vi "MaxEye_ATE_Save_Configuration to File.vi"(0 "file path (use dialog)":path, 5 "Variant":variant, 7 "Config Header":string, 11 "error in (no error)":errorcluster) -> (15 "error out":errorcluster)   [LabVIEW 2021]
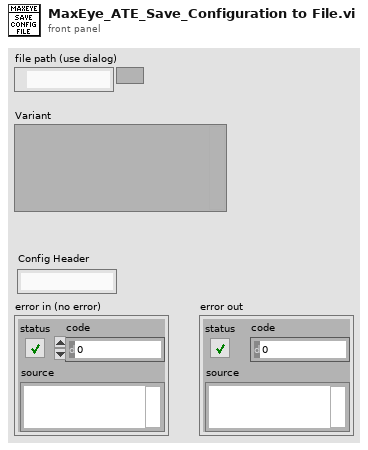
[diagram p1: front panel]
types:
  T1 = enum16{"open", "replace", "create", "open or create", "replace or create", "replace or create with confirmation"}
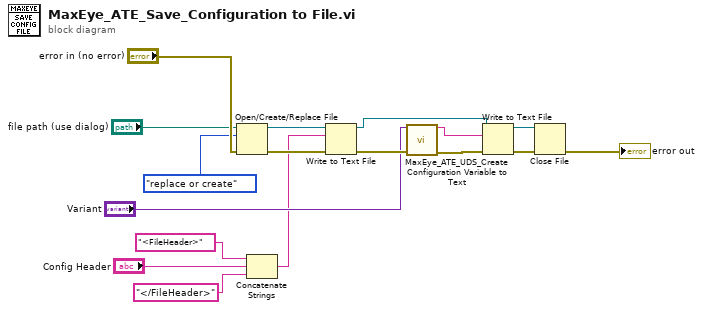
[diagram p0: block diagram]
diagram:
  n1 = Open/Create/Replace File(file path (use dialog)="file path (use dialog)", error in="error in (no error)", operation (0:open)=T1."replace or create") -> (refnum out=w8:refnum<file>, error out=w7:errorcluster)  [unwired: 3 in, 1 out]
  n2 = Concatenate Strings("<FileHeader>" ("string"), "Config Header", "</FileHeader>" ("string")) -> (w3:string)
  n3 = Write to Text File(file (use dialog)=w8, text=w3, error in=w7) -> (refnum out=w4:refnum<file>, error out=w6:errorcluster)  [unwired: 1 in, 1 out]
  n4 = call "MaxEye_ATE_UDS_Create Configuration Variable to Text.vi"("Variant"="Variant", "error in (no error)"=w6) -> ("concatenated string"=w14:string, "error out"=w13:errorcluster)  [unwired: 12 in]
  n5 = Write to Text File(file (use dialog)=w4, text=w14, error in=w13) -> (refnum out=w15:refnum<file>, error out=w16:errorcluster)  [unwired: 1 in, 1 out]
  n6 = Close File(refnum=w15, error in=w16) -> (error out=→"error out":errorcluster)  [unwired: 1 out]
